vi "Get Tags Data.vi"(11 "Channels":refnum<class "TBM channel.lvclass">[](array[class])) -> (2 "Array":dbl[](array[numeric]), 3 "Array 2":string[](array[string]))   [LabVIEW 2015, in "PID Module tests.lvlib"]
uses:
  PID Module tests.lvlib
  <vilib>/NI/Tag Bus Module Framework/channel/TBM channel.lvclass
  <vilib>/NI/Tag Bus/tag/tag descriptor.lvclass/tag descriptor.ctl
  <vilib>/NI/Tag Bus/tag/default value polymorphs/read default value Double.vi
  <vilib>/NI/Tag Bus/tag/tag descriptor.lvclass
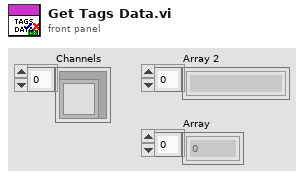
[diagram p1: front panel]
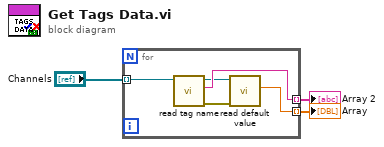
[diagram p0: block diagram]
diagram:
  n1 = for {
    tunnel: "Channels" -> [w8] mode=indexing
    tunnel: [w7] -> w2 mode=indexing
    tunnel: [w4] -> w3 mode=indexing
    n2 = call <vilib>:"read tag name.vi"("system tag in"=w8) -> ("error out"=w6:errorcluster, "name"=w7:string, "system tag out"=w5:refnum<class "TBM channel.lvclass">)  [unwired: 8 in]
    n3 = call-poly <vilib>:"read default value.vi"("error in"=w6, "system tag in"=w5) -> ("default value"=w4:dbl)  [unwired: 6 in, 3 out]
  }
  "Array" <- w3
  "Array 2" <- w2
